vi "Event case-Scrollbar value change.vi"(8 "error in (no error)":errorcluster, 10 "Tick count in":u32, 11 "Queue in":refnum<queue>) -> (0 "error out":errorcluster, 2 "Tick count":u32)   [LabVIEW 2020]
uses:
  Typedefs/Speed Viewer States enum.ctl
  Globals/gl_Time series viewer globals.vi
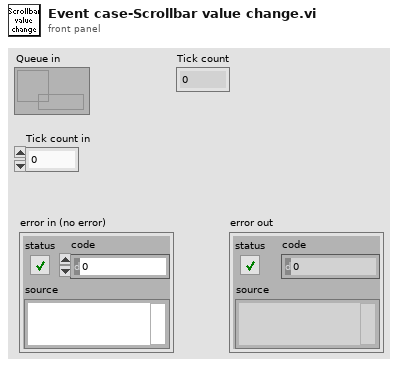
[diagram p1: front panel]
types:
  T1 = typedef "Speed Viewer States enum.ctl" = enum16{"Idle", "Initialise", "Playback", "Scroll bar event", "Speed cursor event", "Back to start", "Exit"}
  T2 = typedef "Time series viewer refs.ctl" = cluster{"This VI":refnum<vi>, "Image control":refnum<vi>, "AVI Mode ind":refnum<vi>, "Play":refnum<vi>, "Stop":refnum<vi>, "Back":refnum<vi>, "Scrollbar":refnum<vi>, "Video length info":refnum<vi>, "Expected speed values":refnum<vi>, "Intensity":refnum<vi>, "Path":refnum<vi>, "Selection sliders":refnum<vi>, "Speed Graph ref":refnum<vi>, "Frame rate set (fps)":refnum<vi>, "Number of rows to generate":refnum<vi>, "VL Image Array":refnum<vi>, "Image Scrollbar":refnum<vi>, "Channel to load":refnum<vi>, "Colour":refnum<vi>}
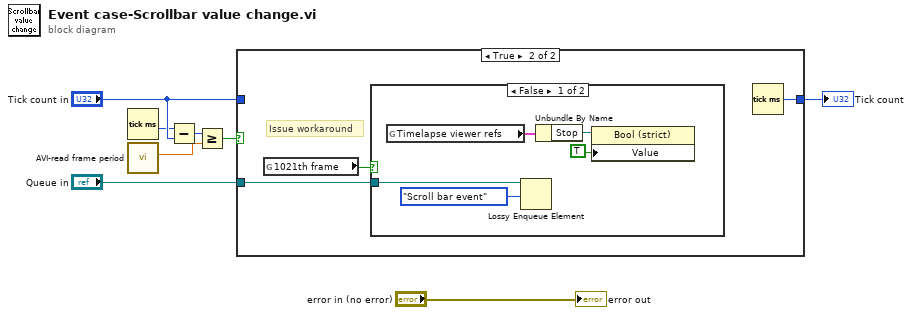
[diagram p0: block diagram]
diagram:
  n1 = Tick Count (ms)() -> (millisecond timer value=w2:u32)
  n2 = call "AVI-read frame period.vi"() -> ("Frame period (ms)"=w8:dbl)  [unwired: 10 in, 1 out]
  n3 = Subtract(x=w2, y="Tick count in") -> (x-y=w3:u32)
  n4 = Greater Or Equal?(x=w3, y=w8) -> (x >= y?=w4:bool)
  n5 = case shown="True" w4 {
    tunnel: [w9 w12] -> w5
    tunnel: "Tick count in" -> [w9 _]
    tunnel: "Queue in" -> [_ w11]
    frame False {
    }
    frame True {
      # "Issue workaround"
      n6 = global read "gl_Time series viewer globals.vi" "1021th frame"() -> (w10:bool)
      n7 = case shown="False" w10 {
        tunnel: w11 -> [w17 _]
        frame False {
          n8 = global read "gl_Time series viewer globals.vi" "Timelapse viewer refs"() -> (w14:T2)
          n9 = Lossy Enqueue Element(queue=w17, element=Speed_Viewer_States_enum."Scroll bar event" ("States")) -> ()  [unwired: 1 in, 4 out]
          n10 = Unbundle By Name(w14) -> ("Stop"=w16:refnum<vi>)
          n11 = property class="Bool (strict)"(reference=w16, "Value"=TRUE ("Stop")) -> ()  [unwired: 1 in, 2 out]
        }
        frame True {
          # "Issue workaround case"
        }
      }
      n12 = Tick Count (ms)() -> (millisecond timer value=w12:u32)
    }
  }
  "Tick count" <- w5
  "error out" <- "error in (no error)"
